vi "Deactivate Pumps.vi"(11 "App Data":T1={"Pump Station Controls"={"Lag Pump"=enum."OFF", "Lead Pump"=enum."OFF", "ALARM"=0.0, "LAG"=0.0, "LEAD"=0.0, "STOP"=0.0}, "Pump Indicators"={"Pump Water Level"=0.0, "ALARM"=FALSE, "LAG"=FALSE, "LEAD"=FALSE, "STOP"=FALSE, "PUMP 1 STATE"=FALSE, "PUMP 2 STATE"=FALSE}, "Alarm"=refnum, "Lag Start Time"=timestamp(0 s since 1904-01-01), "Lead Start Time"=timestamp(0 s since 1904-01-01), "Main Q"=refnum} {"Pump Indicators"."Pump Water Level" scale=0.0..4.0}) -> (3 "App Data 2":T1={"Pump Station Controls"={"Lag Pump"=enum."OFF", "Lead Pump"=enum."OFF", "ALARM"=0.0, "LAG"=0.0, "LEAD"=0.0, "STOP"=0.0}, "Pump Indicators"={"Pump Water Level"=0.0, "ALARM"=FALSE, "LAG"=FALSE, "LEAD"=FALSE, "STOP"=FALSE, "PUMP 1 STATE"=FALSE, "PUMP 2 STATE"=FALSE}, "Alarm"=refnum, "Lag Start Time"=timestamp(0 s since 1904-01-01), "Lead Start Time"=timestamp(0 s since 1904-01-01), "Main Q"=refnum} {"Pump Indicators"."Pump Water Level" scale=0.0..4.0})   [LabVIEW 2024]
uses:
  Pump Switch.ctl
  Pump Controls.ctl
  Pump Indicators.ctl
  Q Info.ctl
  App Data.ctl
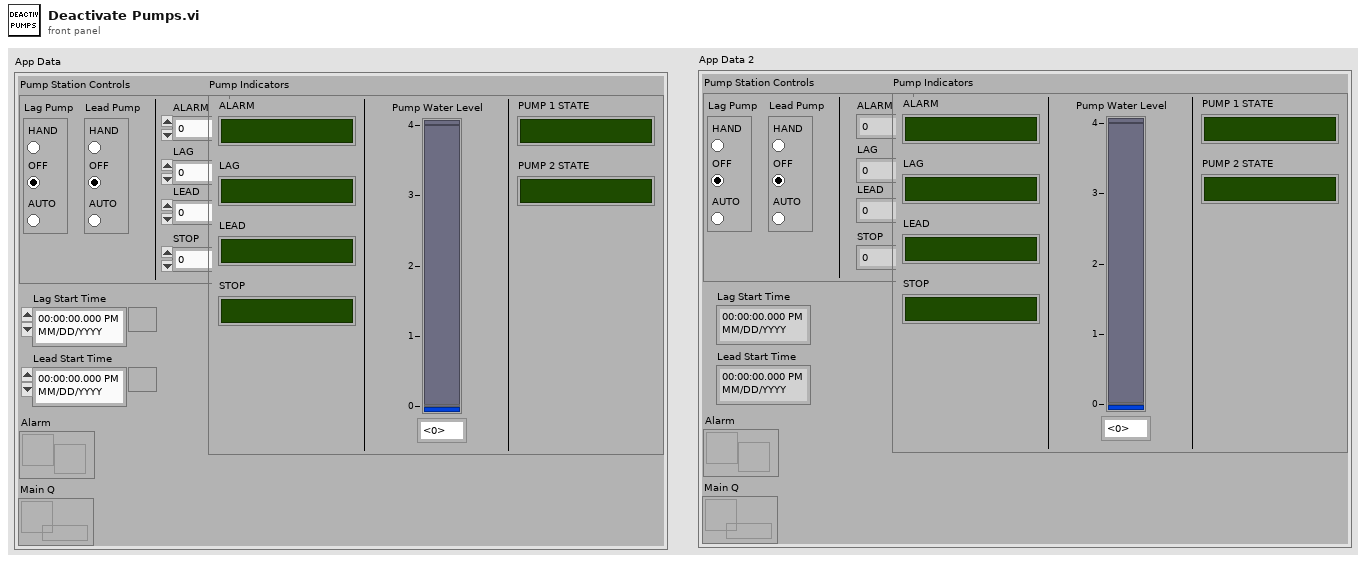
[diagram p1: front panel]
types:
  T1 = typedef "App Data.ctl" = cluster{"Pump Station Controls":T2, "Pump Indicators":T4, "Alarm":refnum<notifier>, "Lag Start Time":timestamp, "Lead Start Time":timestamp, "Main Q":refnum<queue>}
  T2 = typedef "Pump Controls.ctl" = cluster{"Lag Pump":T3, "Lead Pump":T3, "ALARM":dbl, "LAG":dbl, "LEAD":dbl, "STOP":dbl}
  T3 = typedef "Pump Switch.ctl" = enum32{"HAND", "OFF", "AUTO"}
  T4 = typedef "Pump Indicators.ctl" = cluster{"Pump Water Level":dbl, "ALARM":bool, "LAG":bool, "LEAD":bool, "STOP":bool, "PUMP 1 STATE":bool, "PUMP 2 STATE":bool}
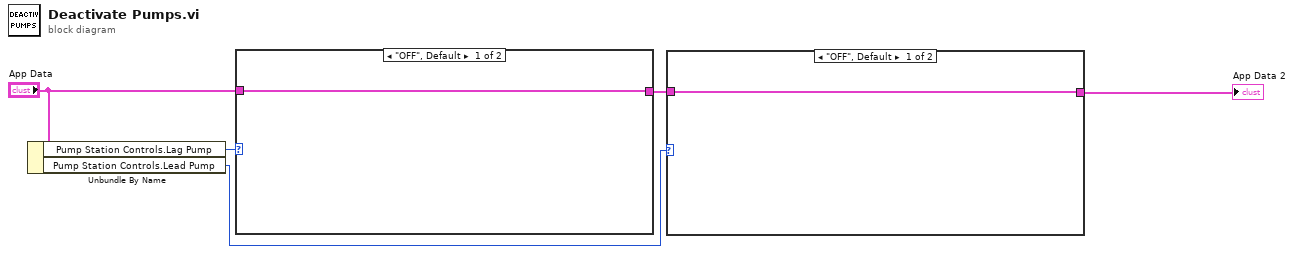
[diagram p0: block diagram]
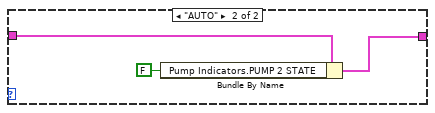
[diagram p2: hidden frame]
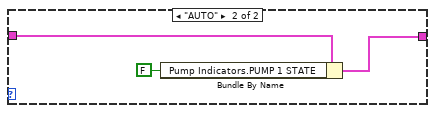
[diagram p3: hidden frame]
diagram:
  n1 = Unbundle By Name("App Data") -> ("Pump Station Controls.Lag Pump"=w5:T3, "Pump Station Controls.Lead Pump"=w2:T3)
  n2 = case shown="\"OFF\", Default" w5 {
    tunnel: "App Data" -> [w6 w9]
    tunnel: [w6 w7] -> w3
    frame "OFF", Default {
    }
    frame "AUTO" {
      n3 = Bundle By Name(cluster=w9, "Pump Indicators.PUMP 1 STATE"=FALSE) -> (w7:T1)
    }
  }
  n4 = case shown="\"OFF\", Default" w2 {
    tunnel: w3 -> [w10 w13]
    tunnel: [w10 w11] -> w1
    frame "OFF", Default {
    }
    frame "AUTO" {
      n5 = Bundle By Name(cluster=w13, "Pump Indicators.PUMP 2 STATE"=FALSE ("Pump Indicators.PUMP 1 STATE")) -> (w11:T1)
    }
  }
  "App Data 2" <- w1
